vi "ClearSurface.vi"(4 "a":sgl, 6 "b":sgl, 8 "No Error":errorcluster, 9 "g":sgl, 10 "r":sgl, 11 "Dst [SDL_Surface *]":i64 format="%.0x") -> (0 "error out":errorcluster)   [LabVIEW 2026, in "SDL3.lvlib" / "Surface.lvlib"]
doc: "<B>Summary</B>\nClear a surface with a specific color, with floating point precision.\n\n<B>Remarks</B>\nThis function handles all surface formats, and ignores any clip rectangle.\n\nIf the surface is YUV, the color is assumed to be in the sRGB colorspace, otherwise the color is assumed to be in the colorspace of the suface."
uses:
  Surface.lvlib
  <vilib>/Utility/error.llb/Error Cluster From Error Code.vi
  Error/Error.lvlib
  Lib/SDL3.dll
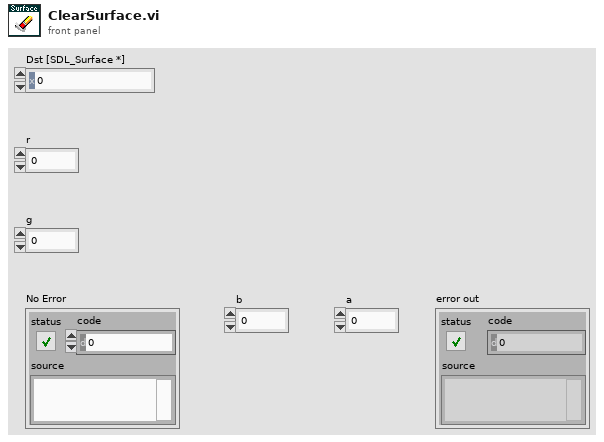
[diagram p1: front panel]
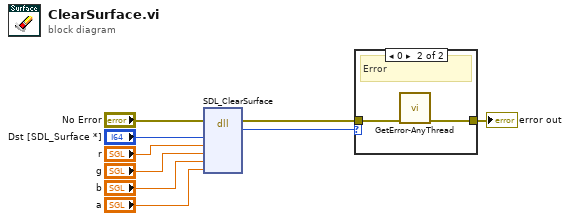
[diagram p0: block diagram]
diagram:
  n1 = dll-call lib="C:/Users/saukko/Dev/LV-SDL3/Sources/SDL3/Lib/SDL3.*" fn="SDL_ClearSurface"(error in="No Error", "surface"="Dst [SDL_Surface *]", "r"="r", "g"="g", "b"="b", "a"="a") -> (error out=w2:errorcluster, "return type"=w1:i32)  [unwired: 7 in, 1 out]
  n2 = case shown="0" w1 {
    tunnel: w2 -> [w10 w12]
    tunnel: [w10 w11] -> w8
    frame Default {
      # "Ok"
    }
    frame 0 {
      # "Error"
      n3 = call "GetError-AnyThread.vi"("No Error"=w12) -> ("Error Out"=w11:errorcluster)  [unwired: 10 in]
    }
  }
  "error out" <- w8
